vi "Config Aout Limit Error.vi"(8 "error in":errorcluster, 9 "Loss (off)":bool, 10 "Capacitance (off)":bool, 11 "VISA resource name":refnum<visa-resource-name>) -> (0 "error out":errorcluster, 3 "VISA resource name out":refnum<visa-resource-name>)   [LabVIEW 2017, in "Andeen-Hagerling 2700.lvlib"]
doc: "The analog outputs levels for the capacitance and loss channels may not exceed the upper and lower voltage protection limits. This VI is used to enable and disable the error reporting associated with this voltage clipping capability."
uses:
  Andeen-Hagerling 2700.lvlib
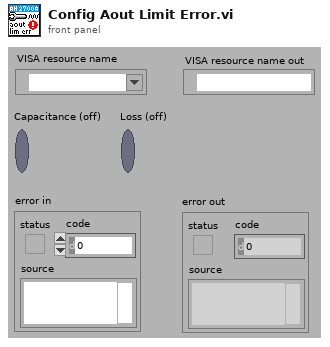
[diagram p1: front panel]
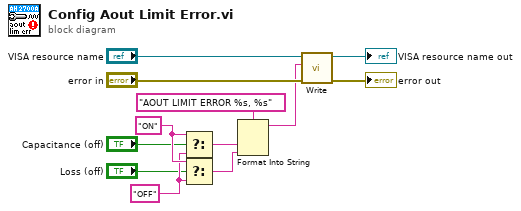
[diagram p0: block diagram]
diagram:
  w7 = "OFF"
  w8 = "ON"
  n1 = Select(t=w8, s="Capacitance (off)", f=w7) -> (s? t:f=w2:string)
  n2 = Select(t=w8, s="Loss (off)", f=w7) -> (s? t:f=w1:string)
  n3 = Format Into String(format string="AOUT LIMIT ERROR %s, %s", w2, w1) -> (resulting string=w3:string)  [unwired: 2 in, 1 out]
  n4 = call "Write.vi"("error in"="error in", "command"=w3, "VISA resource name"="VISA resource name") -> ("error out"=→"error out":errorcluster, "VISA resource name out"=→"VISA resource name out":refnum<visa-resource-name>)  [unwired: 7 in]
